vi "Reset.vi"(8 "error in (no error)":errorcluster, 11 "Debugger in":refnum<class "Debugger.lvclass">) -> (0 "error out":errorcluster, 3 "Debugger out":refnum<class "Debugger.lvclass">)   [LabVIEW 2020, in "Debugger.lvclass"]
uses:
  Debugger.lvclass
  Debugger.lvclass/Debugger.ctl
  Process/Debug Process.lvclass
  C:/Users/anton/Documents/GitHub/triarc-debugger/source/Process/Debug Process.lvclass
  C:/Users/anton/Documents/GitHub/triarc-debugger/source/Debugger/Debugger.lvclass
  C:/Users/anton/Documents/GitHub/triarc-debugger/source/Debug Data Event/Debug Data Listener.lvclass
  Debug Log/Debug Log.lvclass
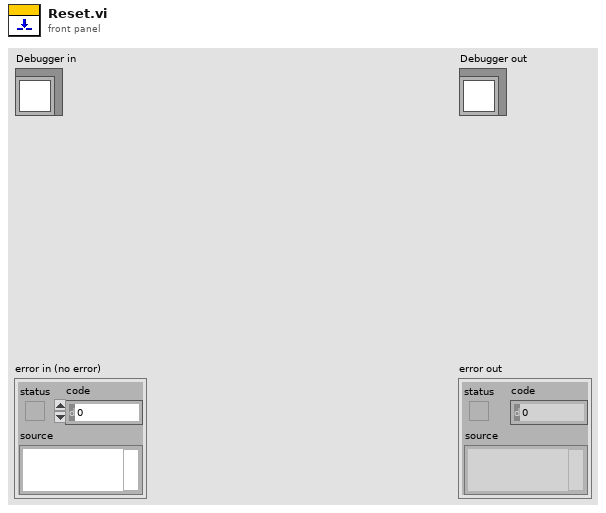
[diagram p1: front panel]
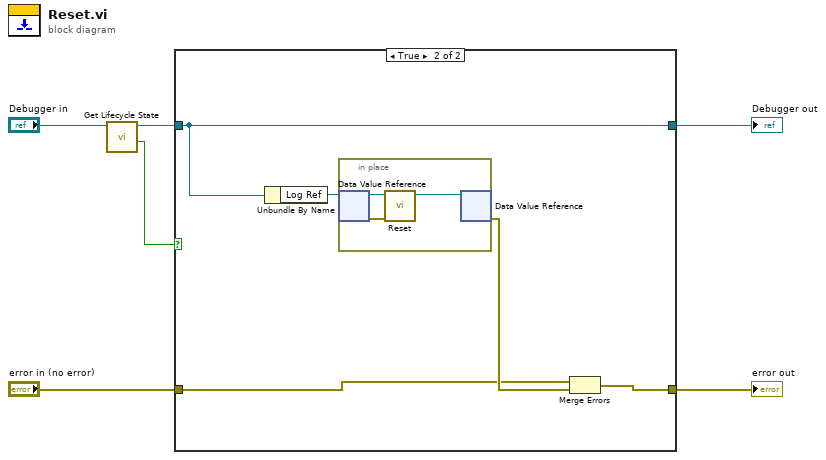
[diagram p0: block diagram]
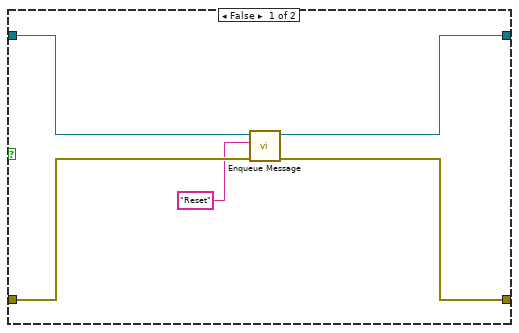
[diagram p2: hidden frame]
diagram:
  n1 = call "Get Lifecycle State.vi"("Process In"="Debugger in") -> ("In Process Loop?"=w1:bool, "Process Out"=w2:refnum<class "Debugger.lvclass">)  [unwired: 7 in, 2 out]
  n2 = case shown="True" w1 {
    tunnel: "error in (no error)" -> [w11 w12]
    tunnel: [w10 w13] -> w5
    tunnel: [w9 w15] -> w4
    tunnel: w2 -> [w7 w15]
    frame False {
      n3 = call "Enqueue Message.vi"("error in (no error)"=w11, "Message"="Reset", "Process In"=w7) -> ("error out"=w10:errorcluster, "Process Out"=w9:refnum<class "Debugger.lvclass">)  [unwired: 7 in]
    }
    frame True {
      n4 = Unbundle By Name(w15) -> ("Log Ref"=w16:refnum<data-value>)
      n5 = in-place {
        n6 = in-place-dvr #1(w16) -> (w19:refnum<class "Debug Log.lvclass">, w18:errorcluster)
        n7 = call "Reset.vi"("error in (no error)"=w18, "Debug Log in"=w19) -> ("Debug Log out"=w17:refnum<class "Debug Log.lvclass">)  [unwired: 8 in, 1 out]
        n8 = in-place-dvr #1(w17) -> (w14:errorcluster)  [unwired: 1 out]
      }
      n9 = Merge Errors(w12, w14) -> (w13:errorcluster)
    }
  }
  "error out" <- w5
  "Debugger out" <- w4
